vi "Instr_InitObject.vi"(8 "error in (no error)":errorcluster, 9 "Instrument Configuration":variant, 10 "Instrument address":refnum<visa-resource-name>, 11 "InstrControl in":refnum<class "InstrControl.lvclass">) -> (0 "error out":errorcluster, 3 "InstrControl out":refnum<class "InstrControl.lvclass">)   [LabVIEW 2013, in "InstrControl.lvclass"]
uses:
  InstrControl.lvclass
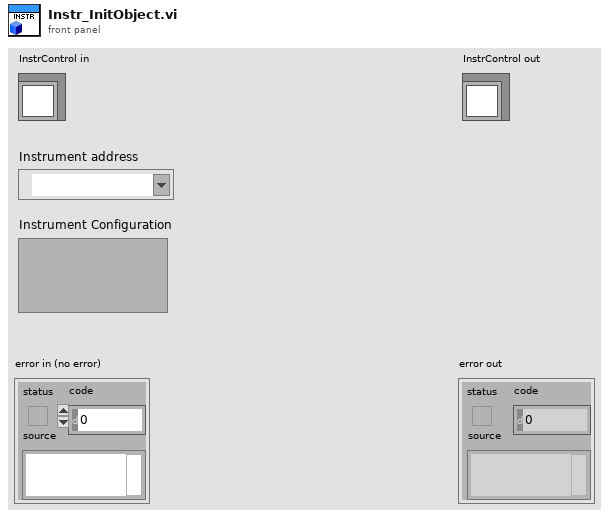
[diagram p1: front panel]
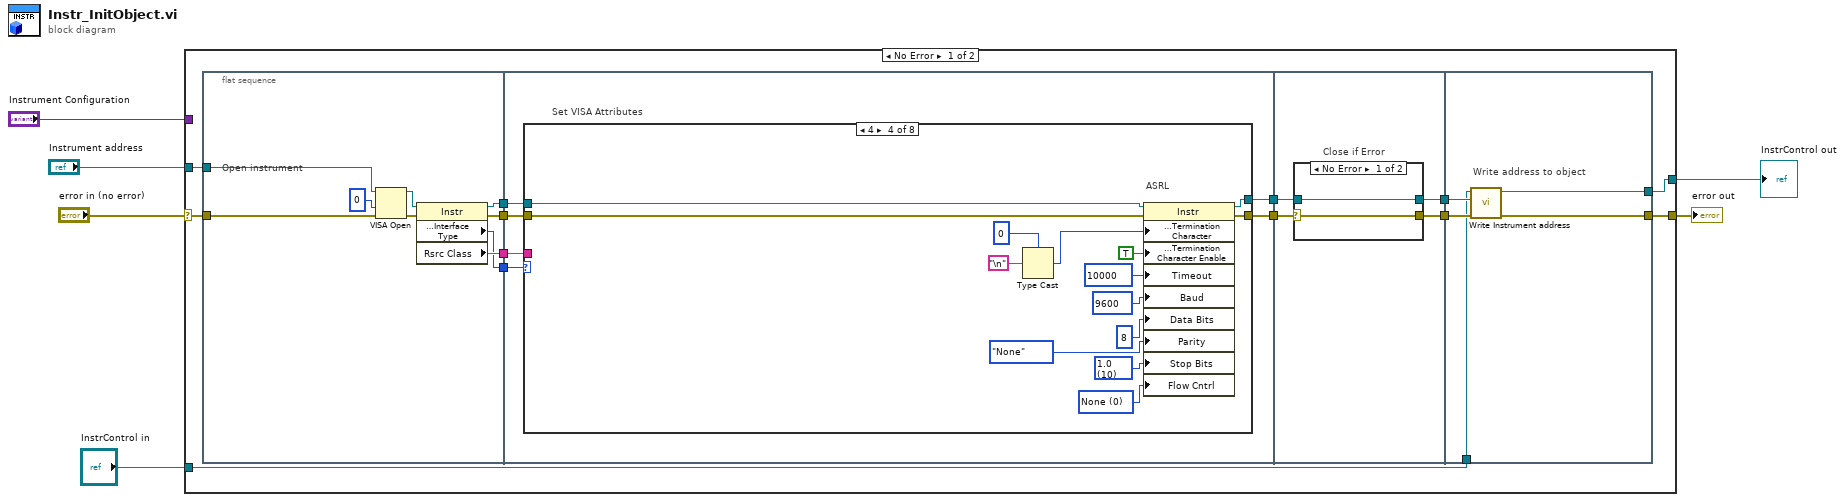
[diagram p0: block diagram]
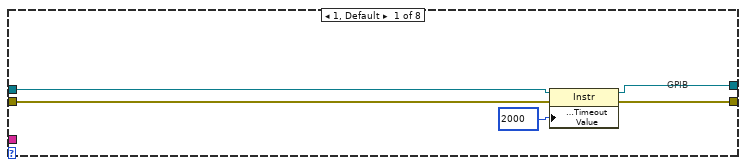
[diagram p2: hidden frame]
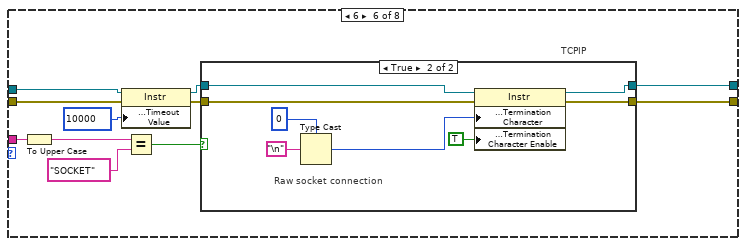
[diagram p6: hidden frame]
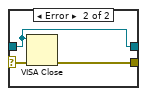
[diagram p10: hidden frame]
diagram:
  n1 = case shown="No Error" "error in (no error)" {
    selector: "error in (no error)" -> [w15 w90]
    tunnel: [w11 w90] -> w5
    tunnel: [w8 w89] -> w3
    tunnel: "InstrControl in" -> [w7 w89]
    tunnel: "Instrument address" -> [w19 _]
    tunnel: "Instrument Configuration" -> [_ _]
    frame No Error {
      n2 = flat-sequence {
        tunnel: w19 -> [w25]
        tunnel: [w24] -> w18
        tunnel: [w23] -> w17
        tunnel: [w22] -> w16
        tunnel: w15 -> [w21]
        tunnel: [w20] -> w14
        tunnel: w18 -> [w34]
        tunnel: w17 -> [w33]
        tunnel: w16 -> [w32]
        tunnel: w14 -> [w31]
        tunnel: [w30] -> w13
        tunnel: [w29] -> w12
        tunnel: w13 -> [w78]
        tunnel: w12 -> [w77]
        tunnel: [w76] -> w10
        tunnel: [w75] -> w9
        tunnel: [w87] -> w11
        tunnel: w10 -> [w88]
        tunnel: w9 -> [w86]
        tunnel: [w85] -> w8
        tunnel: w7 -> [w84]
        frame #0 {
          # "Open instrument"
          n3 = VISA Open(access mode=u32 0, error in (no error)=w21, VISA resource name=w25) -> (VISA resource name=w27:refnum<visa-resource-name>, error out=w28:errorcluster)  [unwired: 2 out]
          n4 = property class="Instr"(reference=w27, error in=w28) -> (reference out=w24:refnum<visa-resource-name>, error out=w20:errorcluster, "Interface Information:Interface Type"=w22:u16, "Rsrc Class"=w23:string)
        }
        frame #1 {
          # "Set VISA Attributes"
          n5 = case shown="4" w32 {
            tunnel: [w37 _ _ w52 _ w64 _ _] -> w29
            tunnel: [w36 _ _ w51 _ w63 _ _] -> w30
            tunnel: w34 -> [w39 _ _ w50 _ w57 _ _]
            tunnel: w31 -> [w38 _ _ w53 _ w55 _ _]
            tunnel: w33 -> [_ _ _ _ _ w62 _ _]
            frame 1, Default {
              # "GPIB"
              n6 = property class="Instr"(reference=w39, error in=w38, "General Settings:Timeout Value"=u32 2000) -> (reference out=w37:refnum<visa-resource-name>, error out=w36:errorcluster)
            }
            frame 2 {
              # "don't have any instrument with this\nanyone happy to fill this in?"
              # "VXI"
            }
            frame 3 {
              # "don't have any instrument with this\nanyone happy to fill this in?"
              # "GPIB-VXI"
            }
            frame 4 {
              w40 = u16 0 items=["None", "XON/XOFF", "RTS/CTS", "XON/XOFF & RTS/CTS", "DTR/DSR", "XON/XOFF & DTR/DSR"] ("flow control (0:none)")
              w41 = u16 10 items=["1.0"=10, "1.5"=15, "2.0"=20] ("stop bits (10: 1 bit)")
              # "ASRL"
              n7 = Type Cast(type=u8 0, x="\n") -> (*(type *) &x=w46:u8)
              n8 = property class="Instr"(reference=w50, error in=w53, "Message Based Settings:Termination Character"=w46, "Message Based Settings:Termination Character Enable"=TRUE, "Timeout"=u32 10000 ("General Settings:Timeout Value"), "Baud"=u32 9600 ("baud rate (9600)"), "Data Bits"=u16 8 ("data bits (8)"), "Parity"=enum16{"None", "Odd", "Even", "Mark", "Space"}."None" ("parity (0:none)"), "Stop Bits"=w41, "Flow Cntrl"=w40) -> (reference out=w52:refnum<visa-resource-name>, error out=w51:errorcluster)
            }
            frame 5 {
              # "don't have any instrument with this\nanyone happy to fill this in?"
              # "PXI"
            }
            frame 6 {
              # "TCPIP"
              n9 = To Upper Case(1:w62) -> (0:w61:string)
              n10 = property class="Instr"(reference=w57, error in=w55, "General Settings:Timeout Value"=u32 10000) -> (reference out=w56:refnum<visa-resource-name>, error out=w54:errorcluster)
              n11 = Equal?(x=w61, y="SOCKET" ("regular expression")) -> (x = y?=w59:bool)
              n12 = case shown="True" w59 {
                tunnel: w54 -> [w65 w74]
                tunnel: [w66 w73] -> w64
                tunnel: [w65 w72] -> w63
                tunnel: w56 -> [w66 w67]
                frame False {
                  # "VXI-11 connection"
                }
                frame True {
                  # "Raw socket connection"
                  n13 = Type Cast(type=u8 0, x="\n") -> (*(type *) &x=w68:u8)
                  n14 = property class="Instr"(reference=w67, error in=w74, "Message Based Settings:Termination Character"=w68, "Message Based Settings:Termination Character Enable"=TRUE) -> (reference out=w73:refnum<visa-resource-name>, error out=w72:errorcluster)
                }
              }
            }
            frame 7 {
              # "USB"
              # "don't have any instrument with this\nanyone happy to fill this in?"
            }
            frame 9 {
              # "FireWire"
              # "don't have any instrument with this\nanyone happy to fill this in?"
            }
          }
        }
        frame #2 {
          # "Close if Error"
          n15 = case shown="No Error" w78 {
            selector: w78 -> [w80 w83]
            tunnel: w77 -> [w79 w81]
            tunnel: [w80 w82] -> w76
            tunnel: [w79 w81] -> w75
            frame No Error {
            }
            frame Error {
              n16 = VISA Close(VISA resource name=w81, error in (no error)=w83) -> (error out=w82:errorcluster)
            }
          }
        }
        frame #3 {
          # "Write address to object"
          n17 = call-dynamic "Write Instrument address.vi"("error in (no error)"=w88, "VISA address"=w86, "InstControl in"=w84) -> ("error out"=w87:errorcluster, "InstControl out"=w85:refnum<class "InstrControl.lvclass">)  [unwired: 7 in]
        }
      }
    }
    frame Error {
    }
  }
  "error out" <- w5
  "InstrControl out" <- w3
